vi "front_panel_withHF2.vi"() -> ()   [LabVIEW 2015]
panel:
  out "Waveform Chart 2":waveform(dbl)(graph)
  out "Waveform Chart":waveform(dbl)(graph)
  out "command string":string
  out "read buffer":string
  in  "Arduino's port":refnum<visa-resource-name>="COM4"
  in  "COMMAND":bool
  in  "TEMPERATURE":bool
  in  "OFF":bool
  in  "stop":bool
  out "LEDs":T1
  in  "Counter Electrode":T2(radio)
  in  "Reference Electrode":T3(radio)=enum."Electrode 1"
  in  "Working Electrode":T3(radio)=enum."Electrode 1"
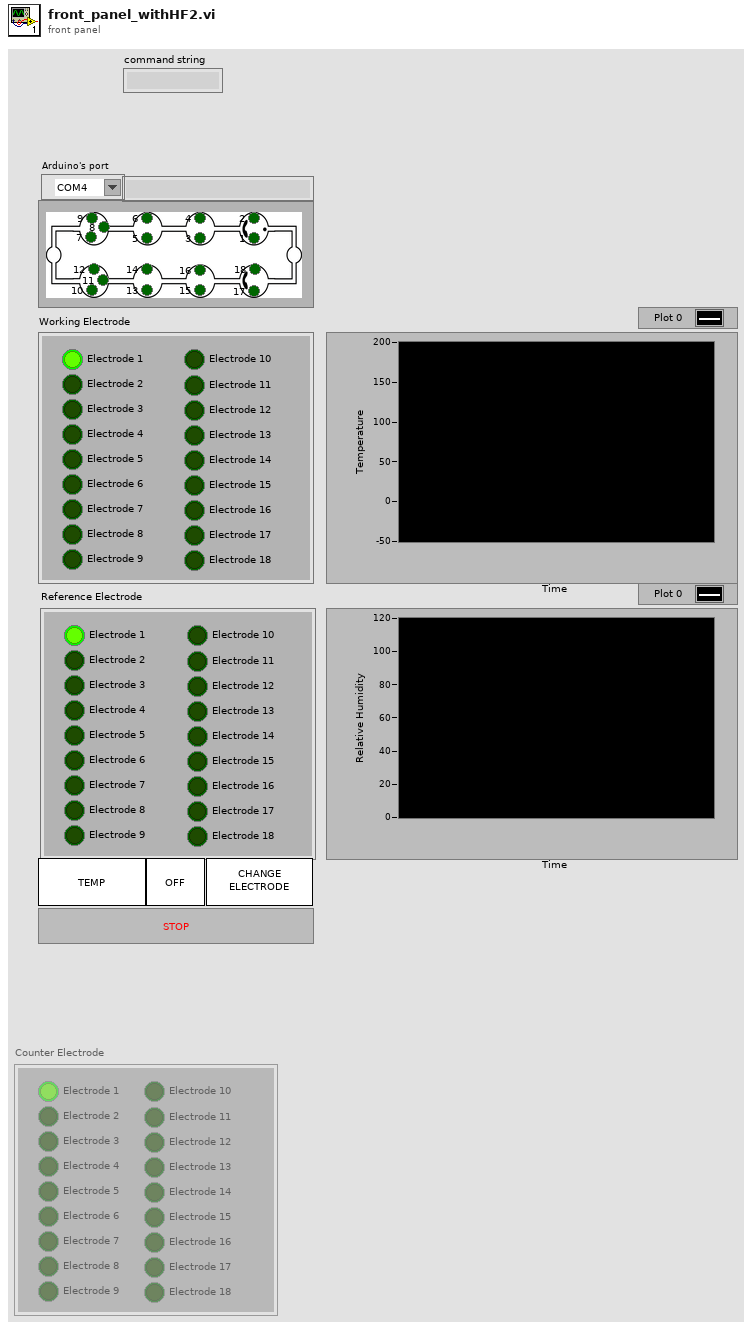
[diagram p1: front panel]
types:
  T1 = cluster{"1":bool, "2":bool, "3":bool, "4":bool, "5":bool, "6":bool, "7":bool, "8":bool, "9":bool, "10":bool, " 11":bool, " 12":bool, "13":bool, "14":bool, "15":bool, "16":bool, "17":bool, "18":bool}
  T2 = enum32{"Electrode 1", "Electrode 2", "Electrode 3", "Electrode 4", "Electrode 5", "Electrode 6", "Electrode 7", "Electrode 8", "Electrode 9", "Electrode 10", "Electrode 11", "Electrode 12", "Electrode 13", "Electrode 14", "Electrode 15", "Electrode 16", "Electrode 17", "Electrode 18"}
  T3 = enum32{"No Selection", "Electrode 1", "Electrode 2", "Electrode 3", "Electrode 4", "Electrode 5", "Electrode 6", "Electrode 7", "Electrode 8", "Electrode 9", "Electrode 10", "Electrode 11", "Electrode 12", "Electrode 13", "Electrode 14", "Electrode 15", "Electrode 16", "Electrode 17", "Electrode 18"}
  T4 = cluster{"VISA resource name out":refnum<visa-resource-name>, "error out":errorcluster}
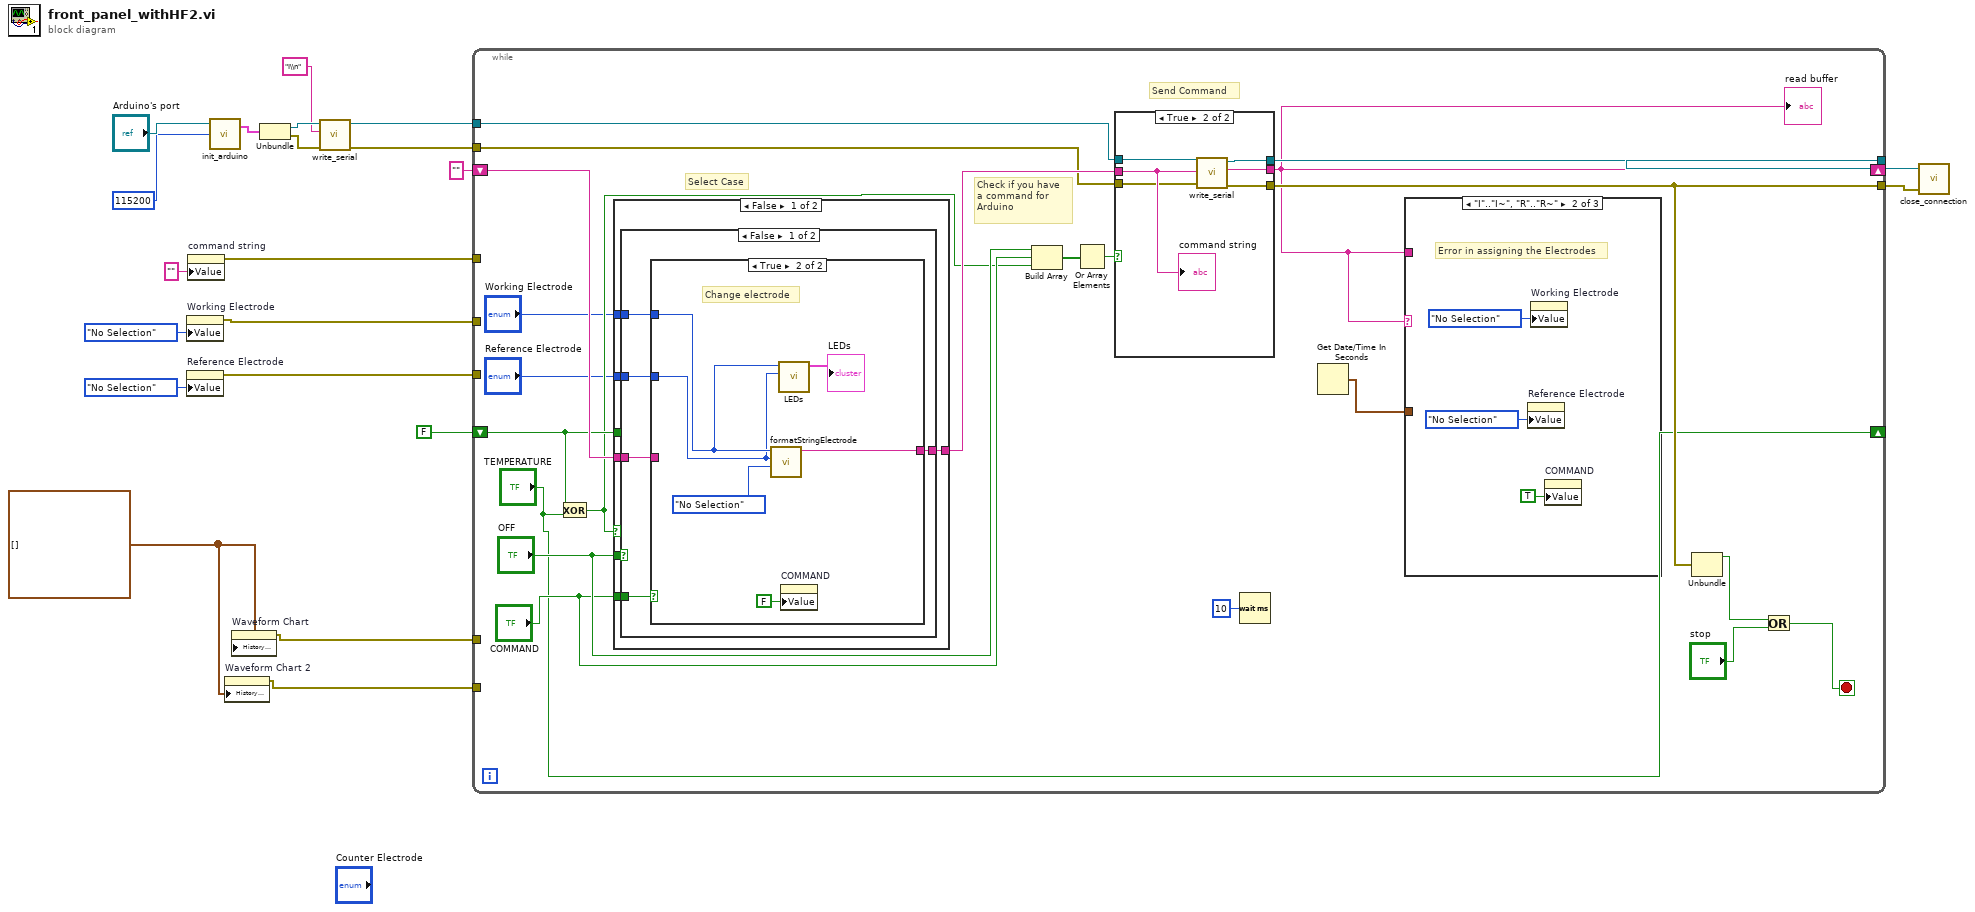
[diagram p0: block diagram]
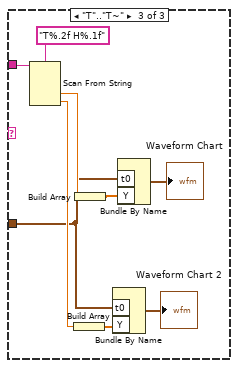
[diagram p3: hidden frame]
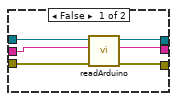
[diagram p4: hidden frame]
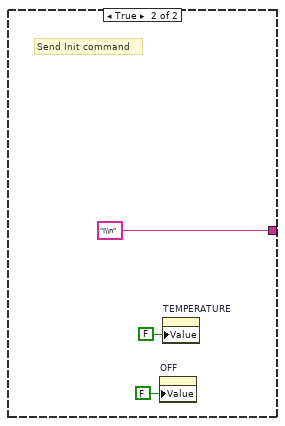
[diagram p6: hidden frame]
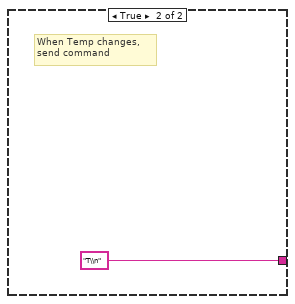
[diagram p7: hidden frame]
diagram:
  w1 = waveform(dbl)[] [] ("History Data")
  n1 = property on="Working Electrode" class="RadioBtnsControl (strict)"("Value"=T3."No Selection" ("Working Electrode")) -> (error out=w7:errorcluster)  [unwired: 2 in, 1 out]
  n2 = property on="Reference Electrode" class="RadioBtnsControl (strict)"("Value"=T3."No Selection" ("Reference Electrode")) -> (error out=w6:errorcluster)  [unwired: 2 in, 1 out]
  n3 = property on="command string" class="Str"("Value"="" ("command string")) -> (error out=w4:errorcluster)  [unwired: 2 in, 1 out]
  n4 = call "init_arduino.vi"("baud rate (9600)"=u32 115200, "Arduino's port"="Arduino's port") -> ("output cluster"=w15:T4)  [unwired: 3 in]
  n5 = property on="Waveform Chart 2" class="WFChart (strict)"("History Data"=w1) -> (error out=w2:errorcluster)  [unwired: 2 in, 1 out]
  n6 = property on="Waveform Chart" class="WFChart (strict)"("History Data"=w1) -> (error out=w3:errorcluster)  [unwired: 2 in, 1 out]
  n7 = Unbundle(w15) -> ("VISA resource name out"=w14:refnum<visa-resource-name>, "error out"=w13:errorcluster)
  n8 = call "write_serial.vi"("error in (no error)"=w13, "write buffer"="I\\n", "VISA resource name"=w14) -> ("error out"=w11:errorcluster, "VISA resource name out"=w12:refnum<visa-resource-name>)  [unwired: 2 in, 1 out]
  n9 = while {
    shift-right: ["TEMPERATURE"] -> _
    shift-left: FALSE ("TEMPERATURE") -> [w36]
    tunnel: [w41] -> w17
    shift-right: [w27] -> _
    shift-left: "" ("read buffer") -> [w40]
    tunnel: [w32] -> w16
    tunnel: w12 -> [w34]
    tunnel: w11 -> [w33]
    tunnel: w7 -> [_]
    tunnel: w6 -> [_]
    tunnel: w4 -> [_]
    tunnel: w3 -> [_]
    tunnel: w2 -> [_]
    stop <- w29 stop-if-true
    # "Send Command"
    # "Check if you have\na command for \nArduino"
    # "Select Case"
    n10 = Exclusive Or(1:"TEMPERATURE", 2:w36) -> (0:w25:bool)
    n11 = case shown="False" w25 {
      tunnel: "OFF" -> [w72 _]
      tunnel: "COMMAND" -> [w71 _]
      tunnel: w36 -> [_ _]
      tunnel: [w70 "T\\n"] -> w42
      tunnel: "Working Electrode" -> [w69 _]
      tunnel: "Reference Electrode" -> [w68 _]
      tunnel: w40 -> [w67 _]
      frame False {
        n12 = case shown="False" w72 {
          tunnel: w71 -> [w77 _]
          tunnel: [w76 "I\\n"] -> w70
          tunnel: w69 -> [w75 _]
          tunnel: w68 -> [w74 _]
          tunnel: w67 -> [w73 _]
          frame False {
            n13 = case shown="True" w77 {
              tunnel: [w78 w83] -> w76
              tunnel: w75 -> [_ w80]
              tunnel: w74 -> [_ w79]
              tunnel: w73 -> [w78 _]
              frame False {
                # "Nothing happens"
              }
              frame True {
                # "Change electrode"
                n14 = call "formatStringElectrode.vi"("Counter Electrode"=T3."No Selection", "Reference Electrode"=w79, "Working Electrode"=w80) -> ("output string"=w83:string)  [unwired: 1 in, 3 out]
                n15 = call "LEDs.vi"("Reference"=w79, "Working"=w80) -> ("Cluster"=→"LEDs":T1)  [unwired: 9 in]
                n16 = property on="COMMAND" class="Bool (strict)"("Value"=FALSE ("COMMAND")) -> ()  [unwired: 2 in, 2 out]
              }
            }
          }
          frame True {
            # "Send Init command"
            n17 = property on="OFF" class="Bool (strict)"("Value"=FALSE ("OFF")) -> ()  [unwired: 2 in, 2 out]
            n18 = property on="TEMPERATURE" class="Bool (strict)"("Value"=FALSE ("TEMPERATURE")) -> ()  [unwired: 2 in, 2 out]
          }
        }
      }
      frame True {
        # "When Temp changes, \nsend command"
      }
    }
    n19 = Build Array("OFF", "COMMAND", w25) -> (w35:bool[])
    n20 = Or Array Elements(Boolean array=w35) -> (logical OR=w39:bool)
    n21 = case shown="True" w39 {
      tunnel: w42 -> [w58 w66]
      tunnel: [w59 w65] -> w27
      tunnel: [w60 w64] -> w41
      tunnel: [w57 w63] -> w32
      tunnel: w34 -> [w56 w62]
      tunnel: w33 -> [w55 w61]
      frame False {
        n22 = call "readArduino.vi"("error in (no error)"=w55, "String"=w58, "reference"=w56) -> ("error out"=w57:errorcluster, "read buffer"=w59:string, "VISA resource name out"=w60:refnum<visa-resource-name>)  [unwired: 6 in]
      }
      frame True {
        n23 = call "write_serial.vi"("error in (no error)"=w61, "write buffer"=w66, "VISA resource name"=w62) -> ("error out"=w63:errorcluster, "read buffer"=w65:string, "VISA resource name out"=w64:refnum<visa-resource-name>)  [unwired: 2 in]
        "command string" <- w66
      }
    }
    "read buffer" <- w27
    n24 = Wait (ms)(milliseconds to wait=u32 10) -> ()  [unwired: 1 out]
    n25 = Get Date/Time In Seconds() -> (seconds since 1Jan1904=w24:timestamp)
    n26 = case shown="\"I\"..\"I~\", \"R\"..\"R~\"" w27 {
      tunnel: w27 -> [_ _ w54]
      tunnel: w24 -> [_ _ w47]
      frame "False", Default {
      }
      frame "I".."I~", "R".."R~" {
        # "Error in assigning the Electrodes"
        n27 = property on="Reference Electrode" class="RadioBtnsControl (strict)"("Value"=T3."No Selection" ("Reference Electrode")) -> ()  [unwired: 2 in, 2 out]
        n28 = property on="Working Electrode" class="RadioBtnsControl (strict)"("Value"=T3."No Selection" ("Working Electrode")) -> ()  [unwired: 2 in, 2 out]
        n29 = property on="COMMAND" class="Bool (strict)"("Value"=TRUE ("COMMAND")) -> ()  [unwired: 2 in, 2 out]
      }
      frame "T".."T~" {
        n30 = Scan From String(format string="T%.2f H%.1f", input string=w54) -> (output 1=w51:dbl, output 2=w49:dbl)  [unwired: 4 in, 3 out]
        n31 = Build Array(w49) -> (w48:dbl[])
        n32 = Build Array(w51) -> (w50:dbl[])
        n33 = Bundle By Name("t0"=w47, "Y"=w48) -> (→"Waveform Chart 2":waveform(dbl))  [unwired: 1 in]
        n34 = Bundle By Name("t0"=w47, "Y"=w50) -> (→"Waveform Chart":waveform(dbl))  [unwired: 1 in]
      }
    }
    n35 = Unbundle(w32) -> ("status"=w31:bool)  [unwired: 2 out]
    n36 = Or(x=w31, y="stop") -> (x .or. y?=w29:bool)
  }
  n37 = call "close_connection.vi"("error in"=w16, "VISA resource name out"=w17) -> ()  [unwired: 1 in, 1 out]
